vi "MFR Flow to SP winMAX.vi"() -> (2 "MFC array":dbl[](array[numeric]))   [LabVIEW 2011]
panel:
  in  "Address":dbl=65.0
  in  "SP":dbl=67.0
  # "0 to 64000"
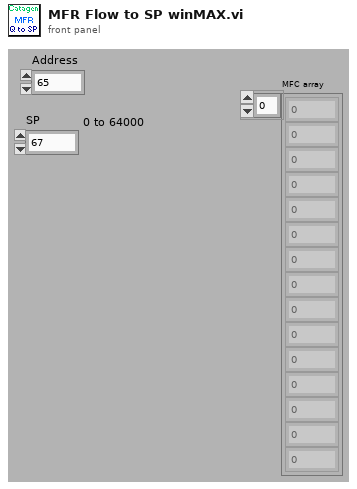
[diagram p1: front panel]
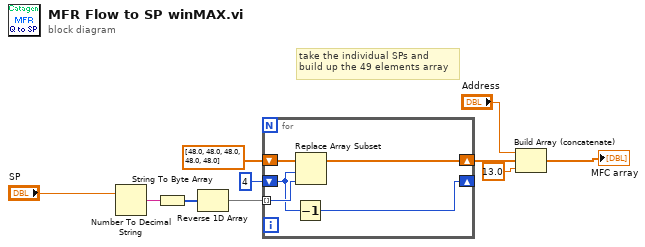
[diagram p0: block diagram]
diagram:
  # "take the individual SPs and \nbuild up the 49 elements array"
  n1 = Number To Decimal String(number="SP") -> (decimal integer string=w6:string)  [unwired: 1 in]
  n2 = String To Byte Array(string=w6) -> (unsigned byte array=w9:u8[])
  n3 = Reverse 1D Array(array=w9) -> (reversed array=w10:u8[])
  n4 = for {
    tunnel: w10 -> [w13] mode=indexing
    shift-right: [w12] -> _
    shift-left: u8 4 -> [w11]
    shift-right: [w14] -> w4
    shift-left: dbl[] [48.0, 48.0, 48.0, 48.0, 48.0] -> [w15]
    n5 = Decrement(x=w11) -> (x-1=w12:u8)
    n6 = Replace Array Subset(array=w15, new element=w13, index=w11) -> (w14:dbl[])
  }
  n7 = Build Array (concatenate)("Address", w4, 13.0) -> (→"MFC array":dbl[])
